vi "Boonton7200_Get_Function_Code.vi"(8 "Error In":errorcluster, 9 "Special Functions":T1, 10 "Data Value":sgl, 11 "IEEE-488 Bus Mnemonics":T2) -> (0 "Error Out":errorcluster, 2 "GPIB code (IEEE-488)":string)   [LabVIEW 2015, in "Boonton7200.lvlib"]
uses:
  Boonton7200.lvlib
  Boonton7200_IEEE-488_Bus_Mnemonics.ctl
  Boonton7200_Special_Function_Codes.ctl
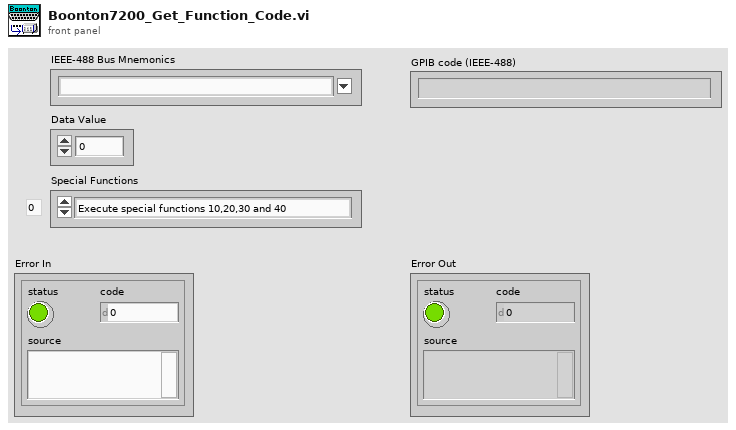
[diagram p1: front panel]
types:
  T1 = typedef "Boonton7200_Special_Function_Codes.ctl" = enum16{"Execute special functions 10,20,30 and 40", "Test Level display and entry", "Capacitance Standard display and entry", "Conductance Standard dispaly and entry", "Capacitance Low Limit display and entry", "Capacitance High Limit dispaly and entry", "IEEE-488 Bus Address display and entry", "End-of-string charecter display and selection", "Capacitance uncertainty display", "Conductance uncertainty dispaly", "Automatic selection(Measurement Ranging Functions)", "Hold current measurement range", "Set and hold 2.000 pF / 2.00 uS range", "Set and hold 20.00 pF / 20.0 uS range", "Set and hold 200.0 pF / 200 uS range", "Set and holde 2000 pF / 2000 uS range", "16 - Not Defined", "17 - Not Defined", "18 - Not Defined", "19 - Not Defined", "Automatic selection(Internal Bias Ranging Functions)", "Hold current bias range", "Set and hold 20.000 V range", "Set and Hold 100.00 V range", "24 - Not Defined", "25 - Not Defined", "26 - Not Defined", "27 - Not Defined", "28 - Not Defined", "29 - Not Defined", "30 Automatic selection(Measurement Filter Functions)", "Filter length = 1 measurement, no average", "Filter length = 2 measurement", "Filter length = 5 measurement", "Filter length = 10 measurement", "Filter length = 20 measurement", "Filter length = 50 measurement", "Filter length = 100 measurement", "Filter length = 200 measurement", "Filter length = 500 measurement", "Normal operation, free-run dispaly(Sercvice Request Functions)", "Disable SRQ interrupt", "Enable SRQ interrupt", "Set SRQ mask when an error occurs", "Set SRQ mask and update dispaly when measurement filter is complete", "Set SRQ mask when capacitance measurement is within the high and low limit settings", "Set SRQ mask when capacitance measurement exceeds the high or low limit settings", "Set SRQ mask when zero or calibration is complete", "Set SRQ mask when sweep is complete", "49 - Not Defined", "Calibrate detector offset(Automatic Calibration and Test Functions)", "Calibrate external bias offset", "Calibrate internal bias offset", "Calibrate full-scale capacitance", "Calibrate conductance phase", "Display internal temperature", "Display amplitude error due to temperature influence", "Display phase error due to temperature influence", "Initialize instrument and erase all program locations", "Initalize software calibration variables"}
  T2 = typedef "Boonton7200_IEEE-488_Bus_Mnemonics.ctl" = string
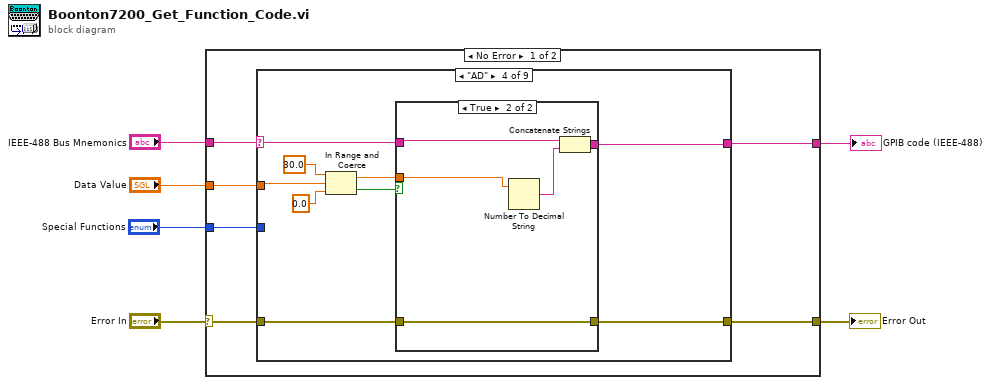
[diagram p0: block diagram]
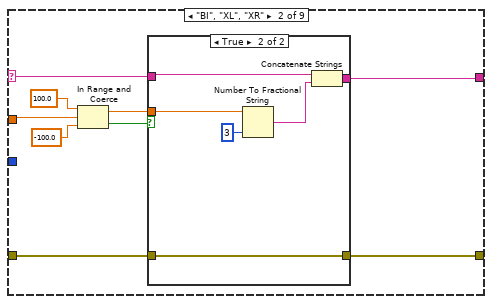
[diagram p3: hidden frame]
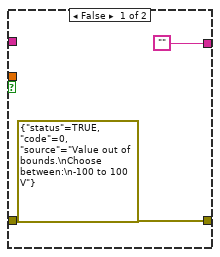
[diagram p4: hidden frame]
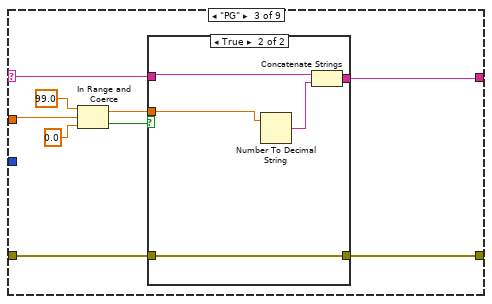
[diagram p5: hidden frame]
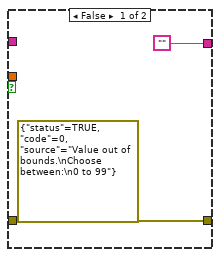
[diagram p6: hidden frame]
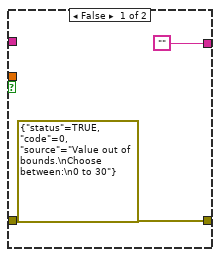
[diagram p7: hidden frame]
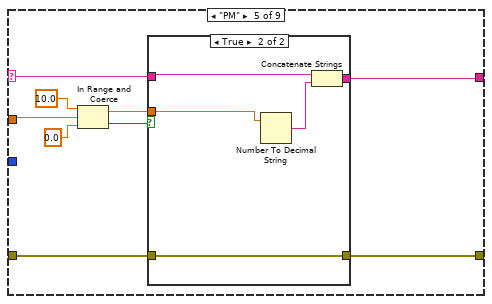
[diagram p8: hidden frame]
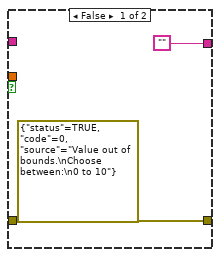
[diagram p9: hidden frame]
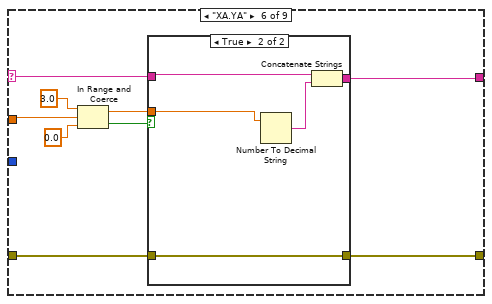
[diagram p10: hidden frame]
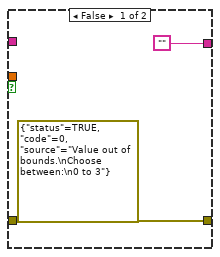
[diagram p11: hidden frame]
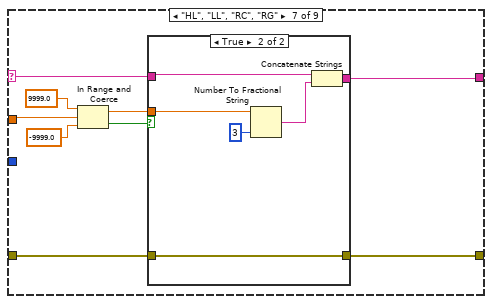
[diagram p12: hidden frame]
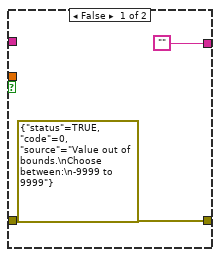
[diagram p13: hidden frame]
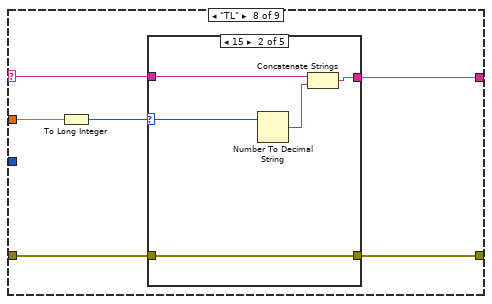
[diagram p14: hidden frame]
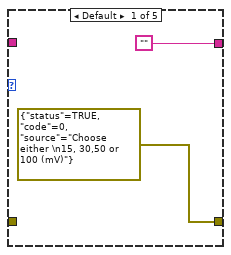
[diagram p15: hidden frame]
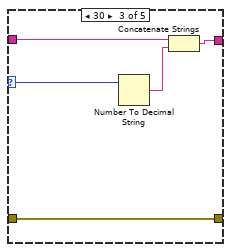
[diagram p16: hidden frame]
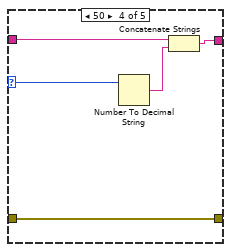
[diagram p17: hidden frame]
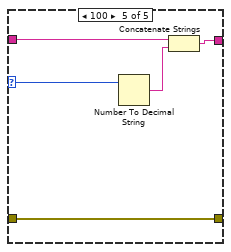
[diagram p18: hidden frame]
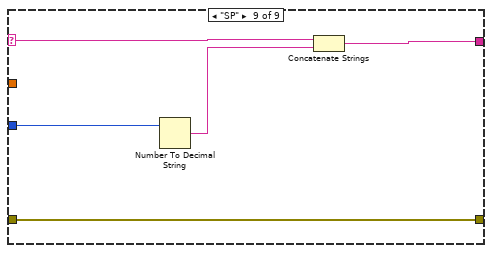
[diagram p19: hidden frame]
diagram:
  n1 = case shown="No Error" "Error In" {
    selector: "Error In" -> [w11 w147]
    tunnel: [w8 w147] -> w5
    tunnel: "IEEE-488 Bus Mnemonics" -> [w12 w146]
    tunnel: [w10 w146] -> w3
    tunnel: "Data Value" -> [w9 _]
    tunnel: "Special Functions" -> [w7 _]
    frame No Error {
      n2 = case shown="\"AD\"" w12 {
        selector: w12 -> [w13 w16 w33 w49 w65 w81 w97 w116 w144]
        tunnel: w11 -> [w14 w23 w40 w56 w72 w88 w104 w118 w141]
        tunnel: [w14 w22 w39 w55 w71 w87 w103 w117 w141] -> w8
        tunnel: [w13 w15 w32 w48 w64 w80 w96 w115 w145] -> w10
        tunnel: w9 -> [_ w21 w38 w54 w70 w86 w102 w113 _]
        tunnel: w7 -> [_ _ _ _ _ _ _ _ w142]
        frame Default {
        }
        frame "BI", "XL", "XR" {
          n3 = In Range and Coerce(upper limit=sgl 100.0, x=w21, lower limit=sgl -100.0) -> (coerced(x)=w17:sgl, In Range?=w18:bool)
          n4 = case shown="True" w18 {
            tunnel: w23 -> [_ w31]
            tunnel: [errorcluster {"status"=TRUE, "code"=0, "source"="Value out of bounds.\nChoose between:\n-100 to 100 V"} ("error constant") w31] -> w22
            tunnel: w17 -> [_ w27]
            tunnel: w16 -> [_ w28]
            tunnel: ["" w29] -> w15
            frame False {
            }
            frame True {
              n5 = Number To Fractional String(number=w27, precision (6)=i16 3) -> (F-format string=w30:string)  [unwired: 2 in]
              n6 = Concatenate Strings(w28, w30) -> (w29:string)
            }
          }
        }
        frame "PG" {
          n7 = In Range and Coerce(upper limit=sgl 99.0, x=w38, lower limit=sgl 0.0) -> (coerced(x)=w34:sgl, In Range?=w35:bool)
          n8 = case shown="True" w35 {
            tunnel: w40 -> [_ w47]
            tunnel: [errorcluster {"status"=TRUE, "code"=0, "source"="Value out of bounds.\nChoose between:\n0 to 99"} ("error constant") w47] -> w39
            tunnel: w34 -> [_ w43]
            tunnel: w33 -> [_ w44]
            tunnel: ["" w45] -> w32
            frame False {
            }
            frame True {
              n9 = Number To Decimal String(number=w43) -> (decimal integer string=w46:string)  [unwired: 1 in]
              n10 = Concatenate Strings(w44, w46) -> (w45:string)
            }
          }
        }
        frame "AD" {
          n11 = In Range and Coerce(upper limit=sgl 30.0, x=w54, lower limit=sgl 0.0) -> (coerced(x)=w50:sgl, In Range?=w51:bool)
          n12 = case shown="True" w51 {
            tunnel: w56 -> [_ w63]
            tunnel: [errorcluster {"status"=TRUE, "code"=0, "source"="Value out of bounds.\nChoose between:\n0 to 30"} ("error constant") w63] -> w55
            tunnel: w50 -> [_ w59]
            tunnel: w49 -> [_ w60]
            tunnel: ["" w61] -> w48
            frame False {
            }
            frame True {
              n13 = Number To Decimal String(number=w59) -> (decimal integer string=w62:string)  [unwired: 1 in]
              n14 = Concatenate Strings(w60, w62) -> (w61:string)
            }
          }
        }
        frame "PM" {
          n15 = In Range and Coerce(upper limit=sgl 10.0, x=w70, lower limit=sgl 0.0) -> (coerced(x)=w66:sgl, In Range?=w67:bool)
          n16 = case shown="True" w67 {
            tunnel: w72 -> [_ w79]
            tunnel: [errorcluster {"status"=TRUE, "code"=0, "source"="Value out of bounds.\nChoose between:\n0 to 10"} ("error constant") w79] -> w71
            tunnel: w66 -> [_ w75]
            tunnel: w65 -> [_ w76]
            tunnel: ["" w77] -> w64
            frame False {
            }
            frame True {
              n17 = Number To Decimal String(number=w75) -> (decimal integer string=w78:string)  [unwired: 1 in]
              n18 = Concatenate Strings(w76, w78) -> (w77:string)
            }
          }
        }
        frame "XA.YA" {
          n19 = In Range and Coerce(upper limit=sgl 3.0, x=w86, lower limit=sgl 0.0) -> (coerced(x)=w82:sgl, In Range?=w83:bool)
          n20 = case shown="True" w83 {
            tunnel: w88 -> [_ w95]
            tunnel: [errorcluster {"status"=TRUE, "code"=0, "source"="Value out of bounds.\nChoose between:\n0 to 3"} ("error constant") w95] -> w87
            tunnel: w82 -> [_ w91]
            tunnel: w81 -> [_ w92]
            tunnel: ["" w93] -> w80
            frame False {
            }
            frame True {
              n21 = Number To Decimal String(number=w91) -> (decimal integer string=w94:string)  [unwired: 1 in]
              n22 = Concatenate Strings(w92, w94) -> (w93:string)
            }
          }
        }
        frame "HL", "LL", "RC", "RG" {
          n23 = In Range and Coerce(upper limit=sgl 9999.0, x=w102, lower limit=sgl -9999.0) -> (coerced(x)=w98:sgl, In Range?=w99:bool)
          n24 = case shown="True" w99 {
            tunnel: w104 -> [_ w112]
            tunnel: [errorcluster {"status"=TRUE, "code"=0, "source"="Value out of bounds.\nChoose between:\n-9999 to 9999"} ("error constant") w112] -> w103
            tunnel: w98 -> [_ w107]
            tunnel: w97 -> [_ w110]
            tunnel: ["" w111] -> w96
            frame False {
            }
            frame True {
              n25 = Number To Fractional String(number=w107, precision (6)=i16 3) -> (F-format string=w108:string)  [unwired: 2 in]
              n26 = Concatenate Strings(w110, w108) -> (w111:string)
            }
          }
        }
        frame "TL" {
          n27 = To Long Integer(number=w113) -> (32bit integer=w114:i32)
          n28 = case shown="15" w114 {
            selector: w114 -> [_ w121 w126 w131 w136]
            tunnel: w118 -> [_ w125 w130 w135 w140]
            tunnel: [errorcluster {"status"=TRUE, "code"=0, "source"="Choose either \n15, 30,50 or 100 (mV)"} ("error constant") w125 w130 w135 w140] -> w117
            tunnel: w116 -> [_ w123 w128 w133 w138]
            tunnel: ["" w124 w129 w134 w139] -> w115
            frame Default {
            }
            frame 15 {
              n29 = Number To Decimal String(number=w121) -> (decimal integer string=w122:string)  [unwired: 1 in]
              n30 = Concatenate Strings(w123, w122) -> (w124:string)
            }
            frame 30 {
              n31 = Number To Decimal String(number=w126) -> (decimal integer string=w127:string)  [unwired: 1 in]
              n32 = Concatenate Strings(w128, w127) -> (w129:string)
            }
            frame 50 {
              n33 = Number To Decimal String(number=w131) -> (decimal integer string=w132:string)  [unwired: 1 in]
              n34 = Concatenate Strings(w133, w132) -> (w134:string)
            }
            frame 100 {
              n35 = Number To Decimal String(number=w136) -> (decimal integer string=w137:string)  [unwired: 1 in]
              n36 = Concatenate Strings(w138, w137) -> (w139:string)
            }
          }
        }
        frame "SP" {
          n37 = Number To Decimal String(number=w142) -> (decimal integer string=w143:string)  [unwired: 1 in]
          n38 = Concatenate Strings(w144, w143) -> (w145:string)
        }
      }
    }
    frame Error {
    }
  }
  "Error Out" <- w5
  "GPIB code (IEEE-488)" <- w3
